vi "Retrieve_GetInstalledSoftware.vi"(8 "error in (no error)":errorcluster, 11 "DevInfo":T1={"Hostname"="", "IPAddress"="", "MAC"="", "SerialNum"="", "Model"="", "Status"="", "FW"="", "OSDesc"="", "ImgTitle"="", "ImgDesc"="", "ImgVer"="", "ImgID"="", "IP Address Request Mode"=1, "SubnetMask"="", "Gateway"="", "DNSServer"=""} {"IP Address Request Mode" items=["Static"=1, "DHCP/Link-Local"=2, "Link-Local Only"=4, "DHCP Only"=8]}) -> (0 "error out":errorcluster, 3 "InstalledSoftware":string[](array[string]))   [LabVIEW 2021]
uses:
  TypeDefs/DevInfo.ctl
  TypeDefs/TargetAccess.ctl
  <vilib>/nisyscfg/Get Installed Components.vi
  <vilib>/nisyscfg/Close (System).vi
  <vilib>/nisyscfg/nisyscfg.lvlib
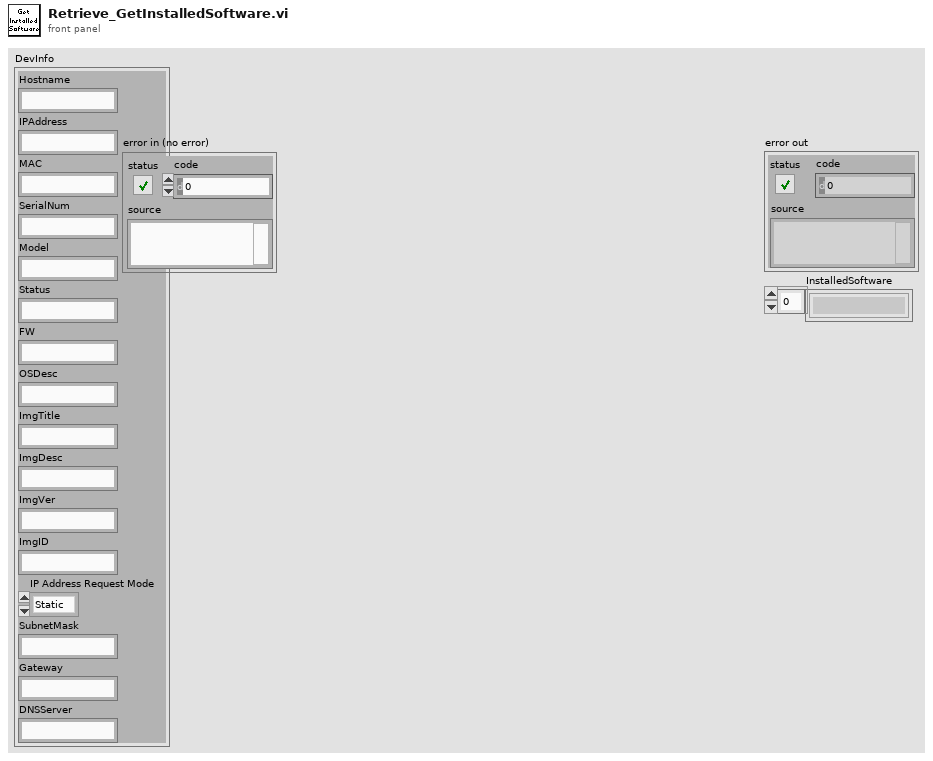
[diagram p1: front panel]
types:
  T1 = typedef "DevInfo.ctl" = cluster{"Hostname":string, "IPAddress":string, "MAC":string, "SerialNum":string, "Model":string, "Status":string, "FW":string, "OSDesc":string, "ImgTitle":string, "ImgDesc":string, "ImgVer":string, "ImgID":string, "IP Address Request Mode":i32, "SubnetMask":string, "Gateway":string, "DNSServer":string}
  T2 = typedef "TargetAccess.ctl" = enum16{"Read-Only", "Admin"}
  T3 = typedef "nisyscfg.lvlib/Software 1.2.ctl" = cluster{"title":string, "description":string, "ID":string, "version":string, "component type":T4}
  T4 = typedef "nisyscfg.lvlib/Component Type.ctl" = u32
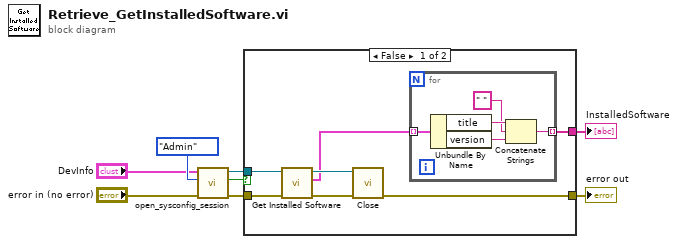
[diagram p0: block diagram]
diagram:
  n1 = call "open_sysconfig_session.vi"("error in (no error)"="error in (no error)", "Target Access"=TargetAccess."Admin", "DevInfo"="DevInfo") -> ("error out"=w4:errorcluster, "Cancelled"=w5:bool, "Session Out"=w6:refnum<k21>)  [unwired: 6 in]
  n2 = case shown="False" w5 {
    tunnel: [w13 w21] -> w2
    tunnel: [w11 _] -> w1
    tunnel: w6 -> [w10 _]
    tunnel: w4 -> [w9 w21]
    frame False {
      n3 = call-poly <vilib>:"Get Installed Software.vi"("error in (no error)"=w9, "Session in"=w10) -> ("error out"=w15:errorcluster, "Software Components"=w12:T3[], "Session out"=w14:refnum<k21>)  [unwired: 7 in]
      n4 = call-poly <vilib>:"Close.vi"("error in (no error)"=w15, "Session in"=w14) -> ("error out"=w13:errorcluster)  [unwired: 9 in]
      n5 = for {
        tunnel: w12 -> [w20] mode=indexing
        tunnel: [w16] -> w11 mode=indexing
        n6 = Unbundle By Name(w20) -> ("title"=w19:string, "version"=w18:string)
        n7 = Concatenate Strings(w19, " " ("string"), w18) -> (w16:string)
      }
    }
    frame True {
    }
  }
  "error out" <- w2
  "InstalledSoftware" <- w1
